vi "Do.vi"(8 "error in (no error)":errorcluster, 10 "Actor in":refnum<class "Actor.lvclass">, 11 "Update_UI Msg":refnum<class "Update_UI Msg.lvclass">) -> (0 "error out":errorcluster, 2 "Actor out":refnum<class "Actor.lvclass">)   [LabVIEW 2025, in "Test_Caller.lvlib" / "Update_UI Msg.lvclass"]
doc: "This VI delivers the message to the actor by calling the appropriate method(s) on the actor."
uses:
  Update_UI Msg.lvclass
  Update_UI Msg.lvclass/Update_UI Msg.ctl
  C:/Users/halstead_rideriver/Documents/Labview_Practice/ATM_Machine_Actor Framework/ATM_ACTORFW/Test_Nested/Test_Nested Messages/New Data Msg/New Data Msg.lvclass
  C:/Program Files (x86)/National Instruments/LabVIEW 2025/vi.lib/ActorFramework/Message/Message.lvclass
  C:/Users/halstead_rideriver/Documents/Labview_Practice/ATM_Machine_Actor Framework/ATM_ACTORFW/Test_Caller/Test_Caller Messages/Update_UI Msg/Update_UI Msg.lvclass
  34700b1e-4b1b-4205-ab4b-28631ba2a4c6.vi
  Test_Caller/Test_Caller.lvclass
  Test_Nested/Test_Nested Messages/New Data Msg/New Data Msg.lvclass
  <vilib>/ActorFramework/Actor/Actor.lvclass
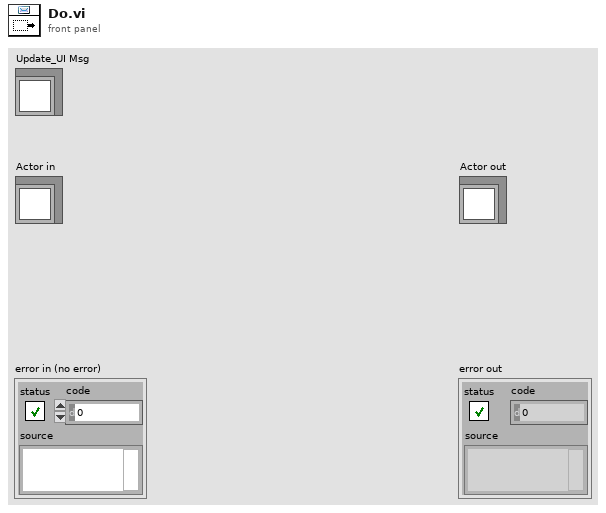
[diagram p1: front panel]
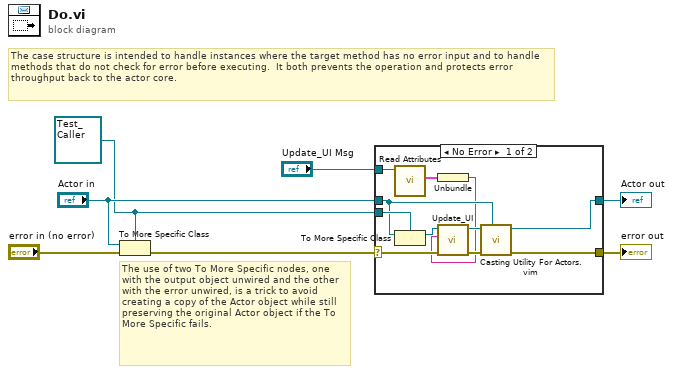
[diagram p0: block diagram]
diagram:
  w2 = refnum<class "Test_Caller.lvclass"> refnum ("Actor in")
  # "The use of two To More Specific nodes, one with the output object unwired and the other with the error unwired, is a trick to avoid creating a copy of the Actor object while still preserving the original Actor object if the To More Specific fails."
  # "The case structure is intended to handle instances where the target method has no error input and to handle methods that do not check for error before executing.  It both prevents the operation and protects error throughput back to the actor core."
  n1 = To More Specific Class(target class=w2, reference="Actor in", error in="error in (no error)") -> (error out=w6:errorcluster)  [unwired: 1 out]
  n2 = case shown="No Error" w6 {
    selector: w6 -> [w18 w20]
    tunnel: [w10 w20] -> w5
    tunnel: [w9 w19] -> w4
    tunnel: "Actor in" -> [w13 w19]
    tunnel: w2 -> [w14 _]
    tunnel: "Update_UI Msg" -> [w15 _]
    frame No Error {
      n3 = call "Read Attributes.vi"("New Data Msg"=w15) -> ("Payload"=w16:cluster{"Data":string})  [unwired: 10 in]
      n4 = To More Specific Class(target class=w14, reference=w13) -> (specific class reference=w17:refnum<class "Test_Caller.lvclass">)  [unwired: 1 in, 1 out]
      n5 = Unbundle(w16) -> ("Data"=w8:string)
      n6 = call-dynamic "Update_UI.vi"("error in (no error)"=w18, "data received"=w8, "Test_Caller in"=w17) -> ("error out"=w11:errorcluster, "Test_Caller out"=w12:refnum<class "Test_Caller.lvclass">)  [unwired: 7 in]
      n7 = call "Casting Utility For Actors.vim"("type"=w13, "error in (no error)"=w11, "Actor in"=w12) -> ("error out"=w10:errorcluster, "Actor out"=w9:refnum<class "Actor.lvclass">)  [unwired: 7 in]
    }
    frame Error {
      # "If type check fails, pass the original object out again."
    }
  }
  "error out" <- w5
  "Actor out" <- w4
